vi "Ritter Reset Meter.vi"(8 "error in (no error)":errorcluster, 11 "VISA resource name":refnum<visa-resource-name>) -> (0 "error out":errorcluster, 2 "Type+Status":string, 3 "VISA resource name Output":refnum<visa-resource-name>)   [LabVIEW 2016]
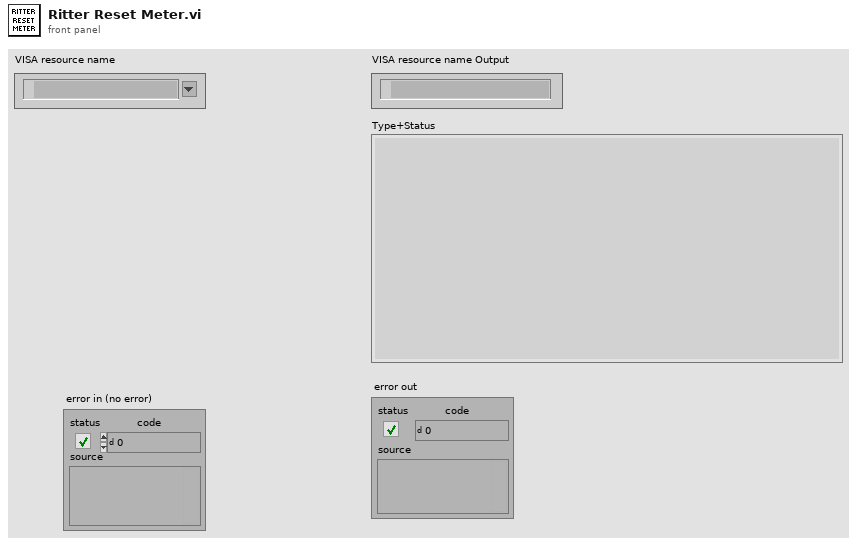
[diagram p1: front panel]
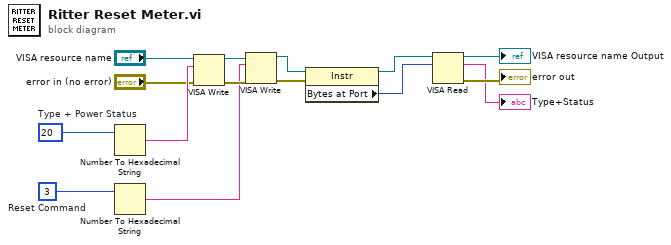
[diagram p0: block diagram]
diagram:
  w14 = u8 20  # Type + Power Status
  w15 = u8 3  # Reset Command
  n1 = Number To Hexadecimal String(2:w14) -> (0:w11:string)  [unwired: 1 in]
  n2 = Number To Hexadecimal String(2:w15) -> (0:w10:string)  [unwired: 1 in]
  n3 = VISA Write(VISA resource name="VISA resource name", write buffer=w11, error in (no error)="error in (no error)") -> (VISA resource name out=w13:refnum<visa-resource-name>, error out=w12:errorcluster)  [unwired: 1 out]
  n4 = VISA Write(VISA resource name=w13, write buffer=w10, error in (no error)=w12) -> (VISA resource name out=w3:refnum<visa-resource-name>, error out=w4:errorcluster)  [unwired: 1 out]
  n5 = property class="Instr"(reference=w3, error in=w4) -> (reference out=w2:refnum<visa-resource-name>, "Bytes at Port"=w1:u32)  [unwired: 1 out]
  n6 = VISA Read(VISA resource name=w2, byte count=w1) -> (VISA resource name out=→"VISA resource name Output":refnum<visa-resource-name>, read buffer=→"Type+Status":string, error out=→"error out":errorcluster)  [unwired: 1 in, 1 out]
